vi "FeedbackDecode_HoverElect.vi"(3 "Instance":i32, 4 "Border":dbl, 5 "PicPos":T2={"Left"=0.0, "Top"=0.0, "Width"=200.0, "Height"=200.0}, 6 "MousePos":T1, 7 "Mode":enum16{"Initialize", "Run"}(ring)) -> (0 "Pic":picture, 1 "Elect":i32=1)   [LabVIEW 2020]
uses:
  <vilib>/Utility/miscctls.llb/LVPoint32TypeDef.ctl
  <vilib>/imath/engines/lvmath2/RunTimeEngine/RangeToken/NIMS_Range.vi
  <instcachedir>/0/NIMS_Range_913EBD8295F041DB898D90A83F67761F.lvgen/NIMS_Range_913EBD8295F041DB898D90A83F67761F_000.vi
  <vilib>/imathl/engines/lvmath/Functions/Error Handling/Create Error.vi
  <vilib>/imath/engines/lvmath2/RunTimeEngine/IndexRead/NIMS V(R2).vi
  <instcachedir>/0/NIMS V(R2)_C76619605A0E4E9F8B2FA9389712AC47.lvgen/NIMS V(R2)_C76619605A0E4E9F8B2FA9389712AC47_000.vi
  <vilib>/imath/engines/lvmath2/RunTimeEngine/BuiltInFunctions/meshgrid2d/NIMS_meshgrid2d(V,V).vi
  <instcachedir>/0/NIMS_meshgrid2d(V,V)_3733343E1C554A708015CFB0432C6A59.lvgen/NIMS_meshgrid2d(V,V)_3733343E1C554A708015CFB0432C6A59_000.vi
  <vilib>/imath/engines/lvmath2/RunTimeEngine/ErrorHandling/NIMS_Create Error From Enums.vi
  <vilib>/imath/engines/lvmath2/RunTimeEngine/BuiltInFunctions/rotate90/NIMS_rotate90.vi
  <instcachedir>/0/NIMS_rotate90_7DC1660D109944E092D2EB6E3185A1B6.lvgen/NIMS_rotate90_7DC1660D109944E092D2EB6E3185A1B6_004.vi
  <vilib>/imath/engines/lvmath2/RunTimeEngine/BuiltInFunctions/reshapemx/NIMS_[GV]_reshapemx.vi
  <instcachedir>/0/NIMS_[GV]_reshapemx_116A7F60707440F78CB0D64335A3F73C.lvgen/NIMS_[GV]_reshapemx_116A7F60707440F78CB0D64335A3F73C_000.vi
  <vilib>/imath/engines/lvmath2/RunTimeEngine/RowToken/NIMS_RowToken_CV_CV.vi
  <instcachedir>/0/NIMS_RowToken_CV_CV_E2834F2F68C5494A92C49C498959A73E.lvgen/NIMS_RowToken_CV_CV_E2834F2F68C5494A92C49C498959A73E_000.vi
  <vilib>/imath/engines/lvmath2/RunTimeEngine/RowToken/NIMS_RowToken_M_CV.vi
  <instcachedir>/0/NIMS_RowToken_M_CV_79C297319A314039B767729C6880A213.lvgen/NIMS_RowToken_M_CV_79C297319A314039B767729C6880A213_000.vi
  <vilib>/imath/engines/lvmath2/RunTimeEngine/NodeEndStatement/NIMS_NodeEndStatement_Output.vi
  <instcachedir>/0/NIMS_NodeEndStatement_Output_53EC0D466D134D7ABD903AC30B43404B.lvgen/NIMS_NodeEndStatement_Output_53EC0D466D134D7ABD903AC30B43404B_002.vi
  <vilib>/imath/engines/lvmath2/RunTimeEngine/ErrorHandling/NIMS_Finalize Error.vi
panel:
  in  "A":dbl[][][](array[numeric])
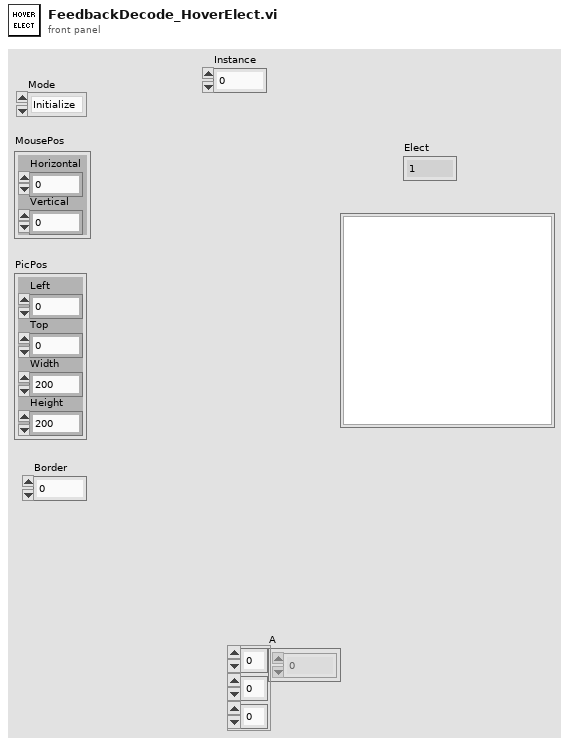
[diagram p1: front panel]
types:
  T1 = typedef "LVPoint32TypeDef.ctl" = cluster{"Horizontal":i32, "Vertical":i32}
  T2 = cluster{"Left":dbl, "Top":dbl, "Width":dbl, "Height":dbl}
  T3 = cluster{"W":dbl, "W":dbl, "Height":dbl, "Width":dbl}
  T4 = cluster{"A[0]":dbl, "A[1]":dbl, "A[2]":dbl, "A[3]":dbl}
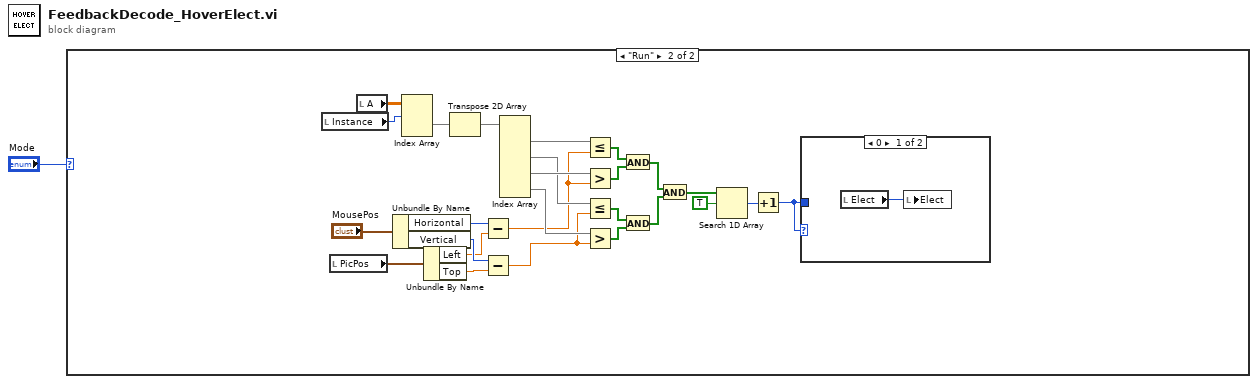
[diagram p0: block diagram]
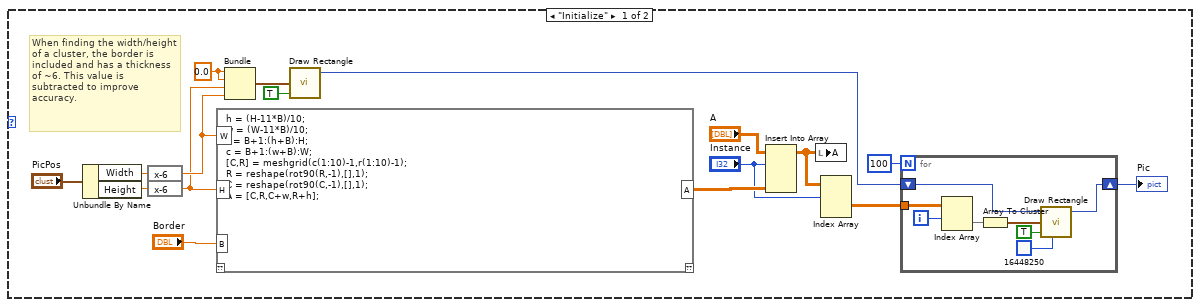
[diagram p2: hidden frame]
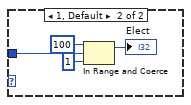
[diagram p3: hidden frame]
diagram:
  n1 = case shown="\"Run\"" "Mode" {
    frame "Initialize" {
      w13 = 0.0 ("W")
      # "When finding the width/height of a cluster, the border is included and has a thickness of ~6. This value is subtracted to improve accuracy."
      n2 = Unbundle By Name("PicPos") -> ("Width"=w10:dbl, "Height"=w8:dbl)
      n3 = expression code="x-6"(w10) -> (w9:dbl)
      n4 = expression code="x-6"(w8) -> (w7:dbl)
      n5 = mathscript code="h = (H-11*B)/10;\nw = (W-11*B)/10;\nr = B+1:(h+B):H;\nc = B+1:(w+B):W;\n[C,R] = meshgrid(c(1:10)-1,r(1:10)-1);\nR = reshape(rot90(R,-1),[],1);\nC = reshape(rot90(C,-1),[],1);\nA = [C,R,C+w,R+h];"("W"=w9, "H"=w7, "B"="Border") -> ("A"=w5:dbl[][])  [unwired: 1 in, 1 out]
      n6 = Bundle("W"=w13, "W"=w13, "Height"=w7, "Width"=w9) -> (w14:T3)  [unwired: 1 in]
      n7 = call <vilib>:"Draw Rectangle.vi"("rect"=w14, "fill?(F)"=TRUE) -> ("new picture"=w18:picture)  [unwired: 7 in]
      n8 = Insert Into Array(array="A", index (dim 0)="Instance", new element=w5) -> (w4:dbl[][][])  [unwired: 2 in]
      n9 = local write "A"(w4) -> ()
      n10 = Index Array(array=w4, index (dim 0)="Instance") -> (element=w3:dbl[][])  [unwired: 2 in]
      n11 = for {
        N: 100 -> [_]
        tunnel: w3 -> [w22]
        shift-right: [w23] -> w11
        shift-left: w18 -> [w24]
        i -> [w20]
        n12 = Index Array(array=w22, index (row)=w20) -> (element=w21:dbl[])  [unwired: 1 in]
        n13 = Array To Cluster(array=w21) -> (cluster=w26:T4)
        n14 = call <vilib>:"Draw Rectangle.vi"("picture"=w24, "rect"=w26, "fill?(F)"=TRUE, "color(black)"=u32 16448250) -> ("new picture"=w23:picture)  [unwired: 5 in]
      }
      "Pic" <- w11
    }
    frame "Run" {
      n15 = local read "Instance"() -> (w226:i32)
      n16 = local read "PicPos"() -> (w230:T2)
      n17 = local read "A"() -> (w228:dbl[][][])
      n18 = Unbundle By Name("MousePos") -> ("Horizontal"=w234:i32, "Vertical"=w236:i32)
      n19 = Index Array(array=w228, index (dim 0)=w226) -> (element=w227:dbl[][])  [unwired: 2 in]
      n20 = Unbundle By Name(w230) -> ("Left"=w235:dbl, "Top"=w237:dbl)
      n21 = Transpose 2D Array(2D array=w227) -> (transposed array=w251:dbl[][])
      n22 = Subtract(x=w234, y=w235) -> (x-y=w233:dbl)
      n23 = Subtract(x=w236, y=w237) -> (x-y=w232:dbl)
      n24 = Index Array(array=w251) -> (element #1=w250:dbl[], element #2=w245:dbl[], element #3=w246:dbl[], element #4=w244:dbl[])  [unwired: 8 in]
      n25 = Less Or Equal?(x=w250, y=w233) -> (x <= y?=w249:bool[])
      n26 = Greater?(x=w246, y=w233) -> (0:w248:bool[])
      n27 = Less Or Equal?(x=w245, y=w232) -> (x <= y?=w242:bool[])
      n28 = Greater?(x=w244, y=w232) -> (0:w243:bool[])
      n29 = And(x=w249, y=w248) -> (x .and. y?=w241:bool[])
      n30 = And(x=w242, y=w243) -> (x .and. y?=w240:bool[])
      n31 = And(x=w241, y=w240) -> (x .and. y?=w239:bool[])
      n32 = Search 1D Array(1D array=w239, element=TRUE) -> (index of element=w238:i32)  [unwired: 1 in]
      n33 = Increment(x=w238) -> (x+1=w229:i32)
      n34 = case shown="0" w229 {
        tunnel: w229 -> [_ w256]
        frame 0 {
          n35 = local read "Elect"() -> (w252:i32)
          n36 = local write "Elect"(w252) -> ()
        }
        frame 1, Default {
          n37 = In Range and Coerce(upper limit=100, x=w256, lower limit=1) -> (coerced(x)=→"Elect":i32)  [unwired: 1 out]
        }
      }
    }
  }
